vi "_deleteConnection.vi"(8 "error in (no error)":errorcluster, 10 "GUID":string, 11 "tWorkerController in":refnum<class "tWorkerController.lvclass">) -> (0 "error out":errorcluster, 1 "Deleted?":bool, 2 "Deleted Connection":T1, 3 "tWorkerController out":refnum<class "tWorkerController.lvclass">)   [LabVIEW 2013, in "tWorkerController.lvlib" / "tWorkerController.lvclass"]
uses:
  tWorkerController.lvclass
  _tcpConnection.ctl
  <vilib>/ActorFramework/Message Enqueuer/Message Enqueuer.lvclass
  tWorkerController.lvclass/tWorkerController.ctl
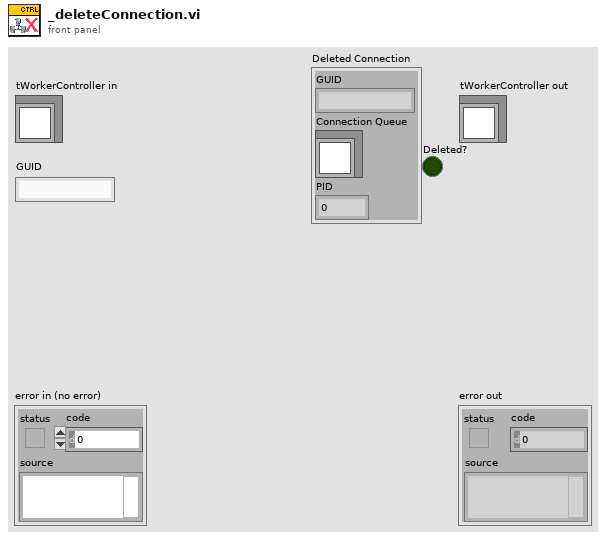
[diagram p1: front panel]
types:
  T1 = typedef "tWorkerController.lvlib/tWorkerController.lvclass/_tcpConnection.ctl" = cluster{"GUID":string, "Connection Queue":refnum<class "Message Enqueuer.lvclass">, "PID":i64}
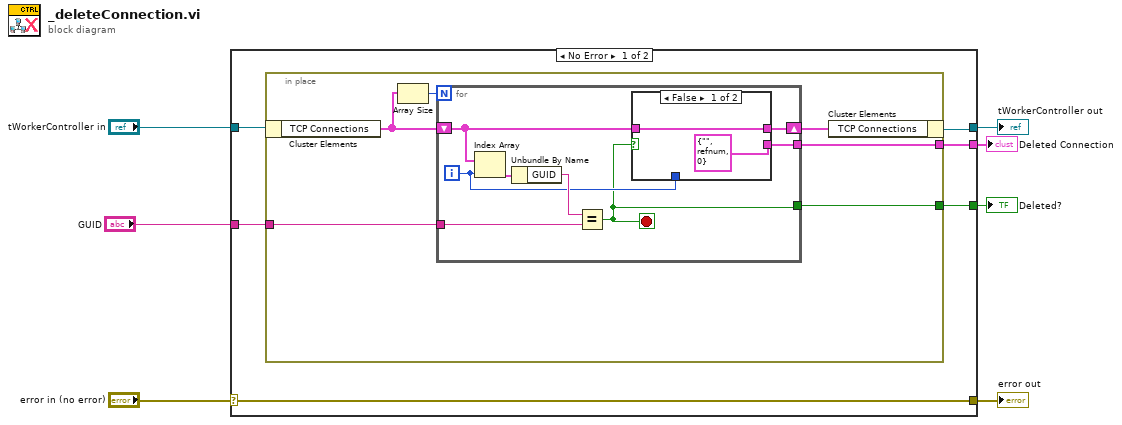
[diagram p0: block diagram]
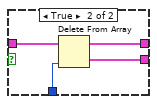
[diagram p2: hidden frame]
diagram:
  n1 = case shown="No Error" "error in (no error)" {
    selector: "error in (no error)" -> [w13 w35]
    tunnel: [w13 w35] -> w6
    tunnel: [w8 w34] -> w4
    tunnel: "tWorkerController in" -> [w12 w34]
    tunnel: "GUID" -> [w11 _]
    tunnel: [w10 _] -> w2
    tunnel: [w9 _] -> w1
    frame No Error {
      n2 = in-place {
        in-place-border: w11 -> [w19]
        in-place-border: [w15] -> w10
        in-place-border: [w14] -> w9
        n3 = in-place-cluster #1(w12) -> ("TCP Connections"=w18:T1[])
        n4 = Array Size(array=w18) -> (size(s)=w17:i32)
        n5 = for {
          N: w17 -> [_]
          tunnel: w19 -> [w25]
          shift-right: [w22] -> w16
          shift-left: w18 -> [w24]
          tunnel: [w21] -> w15
          tunnel: [w20] -> w14
          i -> [w23]
          stop <- w20 stop-if-true
          n6 = Index Array(array=w24, index=w23) -> (element=w27:T1)
          n7 = Unbundle By Name(w27) -> ("GUID"=w26:string)
          n8 = Equal?(x=w26, y=w25) -> (x = y?=w20:bool)
          n9 = case shown="False" w20 {
            tunnel: w24 -> [w29 w33]
            tunnel: w23 -> [_ w32]
            tunnel: [w29 w31] -> w22
            tunnel: [T1 {"GUID"="", "Connection Queue"=refnum, "PID"=0} ("TCP Connection") w30] -> w21
            frame False {
            }
            frame True {
              n10 = Delete From Array(array=w33, index=w32) -> (deleted portion=w30:T1, array with subset deleted=w31:T1[])  [unwired: 1 in]
            }
          }
        }
        n11 = in-place-cluster #1("TCP Connections"=w16) -> (w8:refnum<class "tWorkerController.lvclass">)
      }
    }
    frame Error {
    }
  }
  "error out" <- w6
  "tWorkerController out" <- w4
  "Deleted Connection" <- w2
  "Deleted?" <- w1
